vi "WPI_AnalogTriggerGetOutput.vi"(8 "error in (no error)":errorcluster, 11 "AnalogTriggerDevRef":T1) -> (0 "error out":errorcluster, 1 "Trigger State":bool, 2 "In Window":bool, 3 "AnalogTriggerDevRef":T1)   [LabVIEW 2017]
doc: "Returns the different types of digital output from the trigger.\n\nThis software is licensed. Open the labview\\readme\\WPI Robotics Library Open Source License.txt file for more information."
uses:
  <vilib>/Rock Robotics/SystemInterfaces/AnalogTrigger/FPGA_AnalogTriggerDevRef.ctl
  <vilib>/Rock Robotics/SystemInterfaces/AnalogTrigger/FPGA_AnalogTriggerIndex.ctl
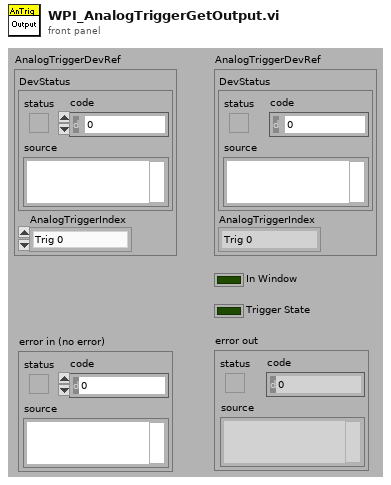
[diagram p1: front panel]
types:
  T1 = typedef "FPGA_AnalogTriggerDevRef.ctl" = cluster{"DevStatus":errorcluster, "AnalogTriggerIndex":T2}
  T2 = typedef "FPGA_AnalogTriggerIndex.ctl" = enum8{"Trig 0", "Trig 1", "Trig 2", "Trig 3", "Trig 4", "Trig 5", "Trig 6", "Trig 7", "Invalid"}
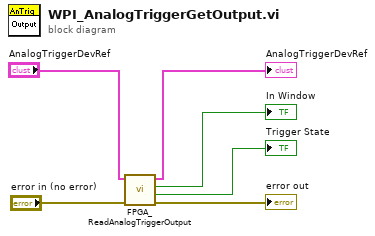
[diagram p0: block diagram]
diagram:
  n1 = call <vilib>:"FPGA_ReadAnalogTriggerOutput.vi"("error in (no error)"="error in (no error)", "AnalogTriggerDevRef"="AnalogTriggerDevRef") -> ("error out"=→"error out":errorcluster, "Trigger State"=→"Trigger State":bool, "In Window"=→"In Window":bool, "AnalogTriggerDevRef"=→"AnalogTriggerDevRef":T1)  [unwired: 6 out]
